vi "Request Refnum.vi"(8 "error in":errorcluster) -> (0 "error out":errorcluster, 3 "Request Refnum":T1)   [LabVIEW 2020, in "SECS Scenarios.lvlib" / "Scenarios Class.lvclass"]
uses:
  Scenarios Class.lvclass
  Request Refnum.ctl
  11-Alarm Management.ctl
  07-Event Report From Equipment.ctl
  14-Process Program Creating Editing or Deleting.ctl
  21-Material Movement.ctl
  23-Equipment Sends Information to Host.ctl
  24-Host Accepts On-Line Request from Equipment.ctl
  25-Host Accepts Off-Line.ctl
  29-Equipment Requests Time Value from Host.ctl
  33-Update Trace Data.ctl
  SECS Communication/S6 Message Class/S6F1.ctl
  SECS Communication/SECS-II Class/Format Code.ctl
  <vilib>/Utility/Data Type/NI_Data Type.lvlib
  SECS Communication/SECS-II Class/SECS-II Class.lvclass
  SECS Communication/S6 Message Class/S6 Message Class.lvclass
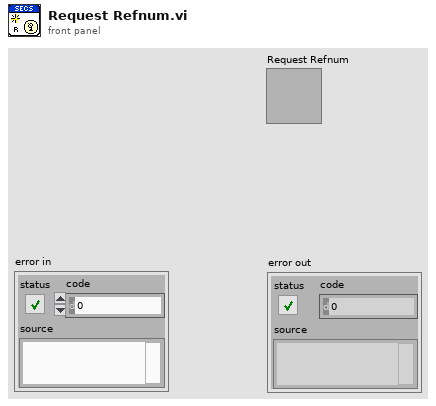
[diagram p1: front panel]
types:
  T1 = typedef "SECS Scenarios.lvlib/Scenarios Class.lvclass/Request Refnum.ctl" = cluster{"11-Alarm Management":refnum<user-event>, "07-Event Report From Equipment":refnum<user-event>, "14-Process Program Creating Editing or Deleting":refnum<user-event>, "21-Material Movement":refnum<user-event>, "23-Equipment Sends Information to Host":refnum<user-event>, "24-Host Accepts On-Line Request from Equipment":refnum<user-event>, "25-Host Refuses On-Line Request":refnum<user-event>, "29-Equipment Requests Time Value from Host":refnum<user-event>, "33-Update Trace Data":refnum<user-event>}
  T2 = typedef "SECS Scenarios.lvlib/Scenarios Class.lvclass/11-Alarm Management.ctl" = cluster{"ALID":u32}
  T3 = typedef "SECS Scenarios.lvlib/Scenarios Class.lvclass/07-Event Report From Equipment.ctl" = cluster{"CEID":u32}
  T4 = typedef "SECS Scenarios.lvlib/Scenarios Class.lvclass/14-Process Program Creating Editing or Deleting.ctl" = cluster{"Process Program CEID":u32}
  T5 = typedef "SECS Scenarios.lvlib/Scenarios Class.lvclass/21-Material Movement.ctl" = cluster{"Material Movement CEID":u32}
  T6 = typedef "SECS Scenarios.lvlib/Scenarios Class.lvclass/23-Equipment Sends Information to Host.ctl" = cluster{"TID":u8, "TEXT":string}
  T7 = typedef "SECS Scenarios.lvlib/Scenarios Class.lvclass/24-Host Accepts On-Line Request from Equipment.ctl" = cluster{"Reply Notifier":refnum<notifier>}
  T8 = typedef "SECS Scenarios.lvlib/Scenarios Class.lvclass/25-Host Accepts Off-Line.ctl" = cluster{"Off-Line":bool}
  T9 = typedef "SECS Scenarios.lvlib/Scenarios Class.lvclass/29-Equipment Requests Time Value from Host.ctl" = cluster{"Reply Notifier":refnum<notifier>}
  T10 = typedef "SECS Scenarios.lvlib/Scenarios Class.lvclass/33-Update Trace Data.ctl" = cluster{"S6F1":T11, "Over":bool}
  T11 = typedef "SECS Communication.lvlib/S6 Message Class.lvclass/S6F1.ctl" = cluster{"TRID":u32, "SMPLN":u32, "STIME":string, "SV":cluster{"Format Code":T12, "Value":variant}[]}
  T12 = typedef "SECS Communication.lvlib/SECS-II Class.lvclass/Format Code.ctl" = enum16{"L", "A", "B", "Boolean", "J", "I1", "I2", "I4", "I8", "U1", "U2", "U4", "U8", "F4", "F8", "Char"}
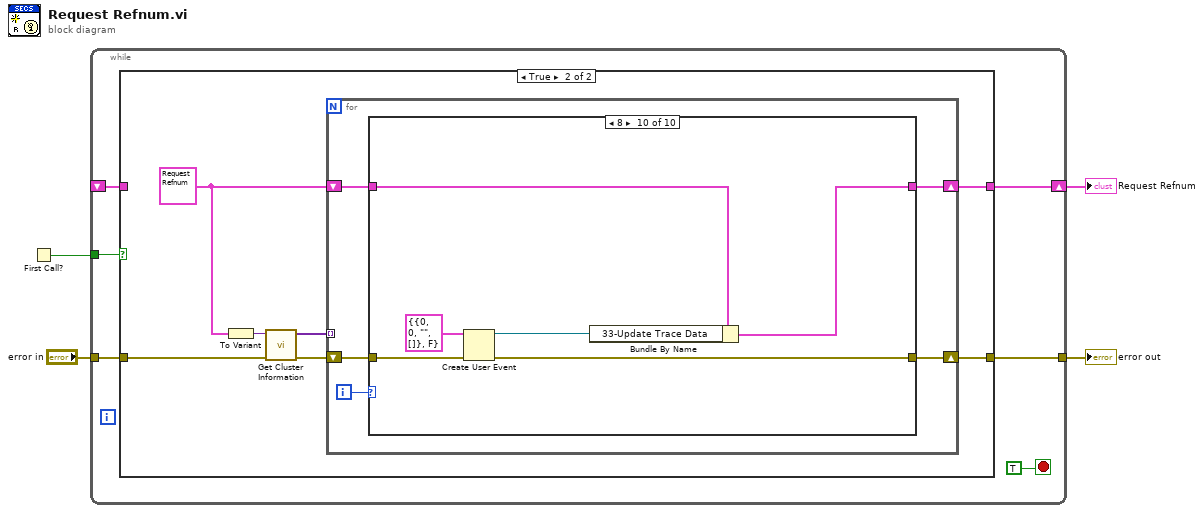
[diagram p0: block diagram]
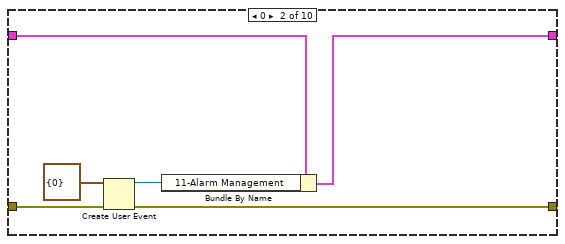
[diagram p4: hidden frame]
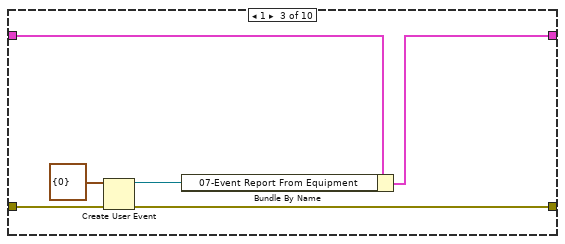
[diagram p5: hidden frame]
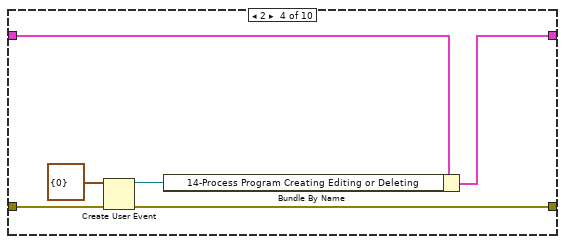
[diagram p6: hidden frame]
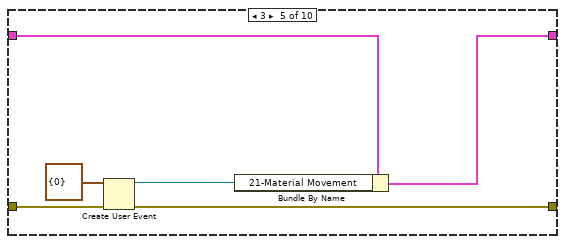
[diagram p7: hidden frame]
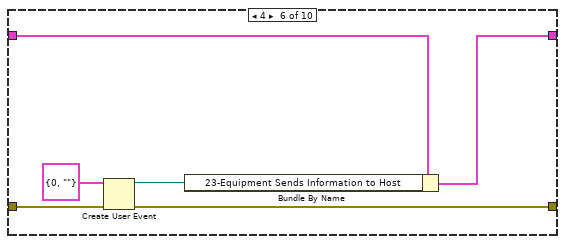
[diagram p8: hidden frame]
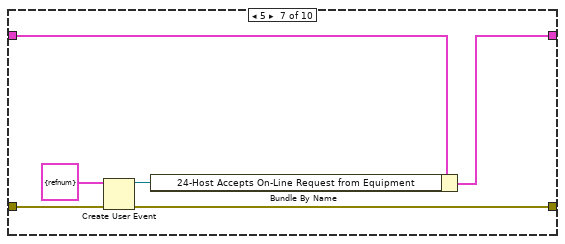
[diagram p9: hidden frame]
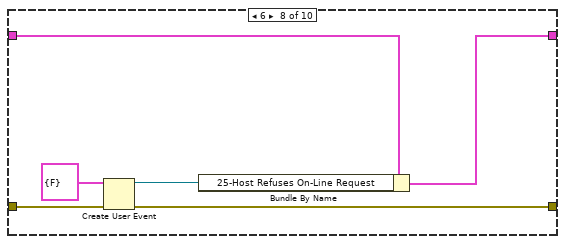
[diagram p10: hidden frame]
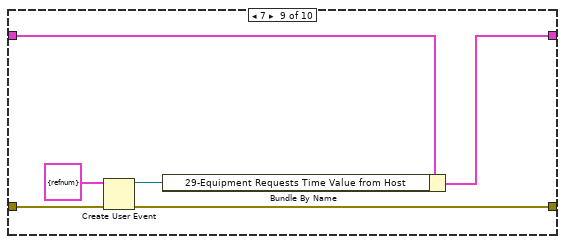
[diagram p11: hidden frame]
diagram:
  n1 = First Call?() -> (First Call?: T/F=w4:bool)
  n2 = while {
    tunnel: "error in" -> [w9]
    tunnel: w4 -> [w10]
    tunnel: [w8] -> w2
    shift-right: [w7] -> w1
    shift-left: _ -> [w6]
    stop <- TRUE stop-if-true
    n3 = case shown="True" w10 {
      tunnel: w9 -> [w11 w18]
      tunnel: [w11 w13] -> w8
      tunnel: [w12 w14] -> w7
      tunnel: w6 -> [w12 _]
      frame False {
      }
      frame True {
        w15 = T1 {"11-Alarm Management"=refnum, "07-Event Report From Equipment"=refnum, "14-Process Program Creating Editing or Deleting"=refnum, "21-Material Movement"=refnum, "23-Equipment Sends Information to Host"=refnum, "24-Host Accepts On-Line Request from Equipment"=refnum, "25-Host Refuses On-Line Request"=refnum, "29-Equipment Requests Time Value from Host"=refnum, "33-Update Trace Data"=refnum} ("Request Refnum")
        n4 = To Variant(anything=w15) -> (Variant=w19:variant)
        n5 = call <vilib>:"Get Cluster Information.vi"("error in (no error)"=w18, "variant"=w19) -> ("error out"=w17:errorcluster, "cluster elements"=w16:variant[])  [unwired: 8 in]
        n6 = for {
          shift-right: [w20] -> w13
          shift-left: w17 -> [w24]
          tunnel: w16 -> [_] mode=indexing
          shift-right: [w21] -> w14
          shift-left: w15 -> [w22]
          i -> [w23]
          n7 = case shown="8" w23 {
            tunnel: w24 -> [w25 w31 w38 w44 w50 w56 w62 w68 w74 w80]
            tunnel: w22 -> [w26 w30 w37 w43 w49 w55 w61 w67 w73 w79]
            tunnel: [w26 w28 w35 w41 w47 w53 w59 w66 w72 w78] -> w21
            tunnel: [w25 w27 w34 w40 w46 w52 w58 w65 w71 w77] -> w20
            frame Default {
            }
            frame 0 {
              n8 = Create User Event(user event datatype=T2 {"ALID"=0} ("11-Alarm Management"), error in=w31) -> (user event=w29:refnum<user-event>, error out=w27:errorcluster)
              n9 = Bundle By Name(cluster=w30, "11-Alarm Management"=w29) -> (w28:T1)
            }
            frame 1 {
              n10 = Create User Event(user event datatype=T3 {"CEID"=0} ("07-Event Report From Equipment"), error in=w38) -> (user event=w36:refnum<user-event>, error out=w34:errorcluster)
              n11 = Bundle By Name(cluster=w37, "07-Event Report From Equipment"=w36) -> (w35:T1)
            }
            frame 2 {
              n12 = Create User Event(user event datatype=T4 {"Process Program CEID"=0} ("14-Process Program Creating Editing or Deleting"), error in=w44) -> (user event=w42:refnum<user-event>, error out=w40:errorcluster)
              n13 = Bundle By Name(cluster=w43, "14-Process Program Creating Editing or Deleting"=w42) -> (w41:T1)
            }
            frame 3 {
              n14 = Create User Event(user event datatype=T5 {"Material Movement CEID"=0} ("21-Material Movement"), error in=w50) -> (user event=w48:refnum<user-event>, error out=w46:errorcluster)
              n15 = Bundle By Name(cluster=w49, "21-Material Movement"=w48) -> (w47:T1)
            }
            frame 4 {
              n16 = Create User Event(user event datatype=T6 {"TID"=0, "TEXT"=""} ("23-Equipment Sends Information to Host"), error in=w56) -> (user event=w54:refnum<user-event>, error out=w52:errorcluster)
              n17 = Bundle By Name(cluster=w55, "23-Equipment Sends Information to Host"=w54) -> (w53:T1)
            }
            frame 5 {
              n18 = Create User Event(user event datatype=T7 {"Reply Notifier"=refnum} ("24-Host Accepts On-Line Request from Equipment"), error in=w62) -> (user event=w60:refnum<user-event>, error out=w58:errorcluster)
              n19 = Bundle By Name(cluster=w61, "24-Host Accepts On-Line Request from Equipment"=w60) -> (w59:T1)
            }
            frame 6 {
              n20 = Create User Event(user event datatype=T8 {"Off-Line"=FALSE} ("25-Host Accepts Off-Line"), error in=w68) -> (user event=w63:refnum<user-event>, error out=w65:errorcluster)
              n21 = Bundle By Name(cluster=w67, "25-Host Refuses On-Line Request"=w63) -> (w66:T1)
            }
            frame 7 {
              n22 = Create User Event(user event datatype=T9 {"Reply Notifier"=refnum} ("29-Equipment Requests Time Value from Host"), error in=w74) -> (user event=w69:refnum<user-event>, error out=w71:errorcluster)
              n23 = Bundle By Name(cluster=w73, "29-Equipment Requests Time Value from Host"=w69) -> (w72:T1)
            }
            frame 8 {
              n24 = Create User Event(user event datatype=T10 {"S6F1"={"TRID"=0, "SMPLN"=0, "STIME"="", "SV"=[]}, "Over"=FALSE} ("33-Update Trace Data"), error in=w80) -> (user event=w75:refnum<user-event>, error out=w77:errorcluster)
              n25 = Bundle By Name(cluster=w79, "33-Update Trace Data"=w75) -> (w78:T1)
            }
          }
        }
      }
    }
  }
  "error out" <- w2
  "Request Refnum" <- w1
